vi "Arduino.vi"() -> ()   [LabVIEW 2015]
uses:
  <vilib>/MakerHub/LINX/Private/Type Defs/User Platform.ctl
  <vilib>/MakerHub/LINX/Private/Type Defs/Interface.ctl
  <vilib>/MakerHub/LINX/Public/Peripherals/PWM/Set Duty Cycle 1 Chan.vi
  <vilib>/MakerHub/LINX/LMH-LINX.lvlib
  <vilib>/MakerHub/LINX/Public/Peripherals/Digital/Digital Write 1 Chan.vi
  <vilib>/MakerHub/LINX/Public/Peripherals/Analog/Analog Read 1 Chan.vi
panel:
  in  "Duty Cycle (0-1)":dbl(knob) scale=0.0..0.2
  out "Loop Rate (Hz) 2":u32
  out "Loop Rate (Hz)":u32
  in  "Serial Port":refnum<visa-resource-name>="N/A"
  in  "Interface":T1
  in  "Platform":T2
  out "Waveform Chart":dbl(graph)
  in  "stop":bool
  in  "PWM Channel":u8
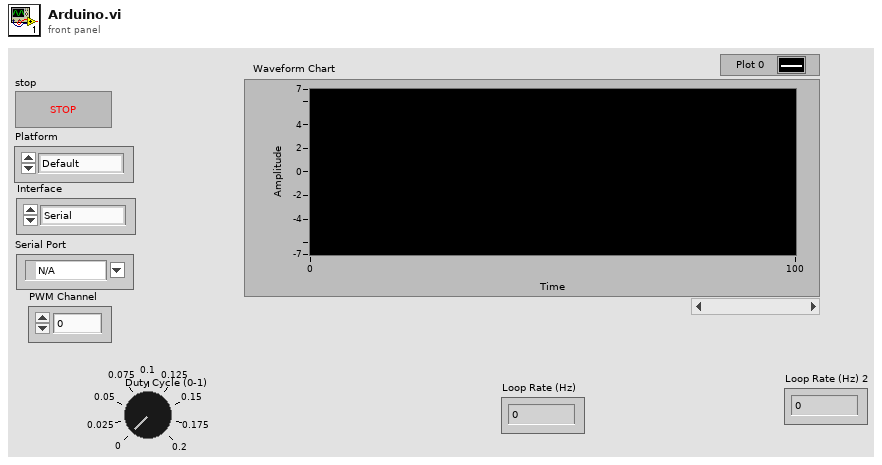
[diagram p1: front panel]
types:
  T1 = typedef "LMH-LINX.lvlib/Interface.ctl" = enum16{"Serial", "TCP"}
  T2 = typedef "LMH-LINX.lvlib/User Platform.ctl" = enum16{"Default", "LINX", "myRIO"}
  T3 = typedef "LMH-LINX.lvlib/LINX Ref.ctl" = cluster{"Platform":T4, "Interface":T1, "LINX Device Config":T5}
  T4 = typedef "LMH-LINX.lvlib/Platform.ctl" = enum16{"LINX", "myRIO"}
  T5 = typedef "LMH-LINX.lvlib/Device.lvlib/LINX Device Config.ctl" = cluster{"Interface":T1, "COM Port":refnum<visa-resource-name>, "TCP Configuration":T6, "Device Family":u8, "Device ID":u8, "Device Name":string, "TCP Ref":refnum<k5>, "Channels":T7}
  T6 = typedef "LMH-LINX.lvlib/Device.lvlib/TCP Config.ctl" = cluster{"IP Address":string, "Port":u16}
  T7 = typedef "LMH-LINX.lvlib/Channels.ctl" = cluster{"DI":u8[], "DO":u8[], "AI":u8[], "AO":u8[], "PWM":u8[], "QE":u8[], "UART":u8[], "I2C 2":u8[], "SPI":u8[], "CAN":u8[], "Servo":u8[], "AI Ref (V)":dbl, "AO Ref (V)":dbl, "AO Resolution (Bits)":u8}
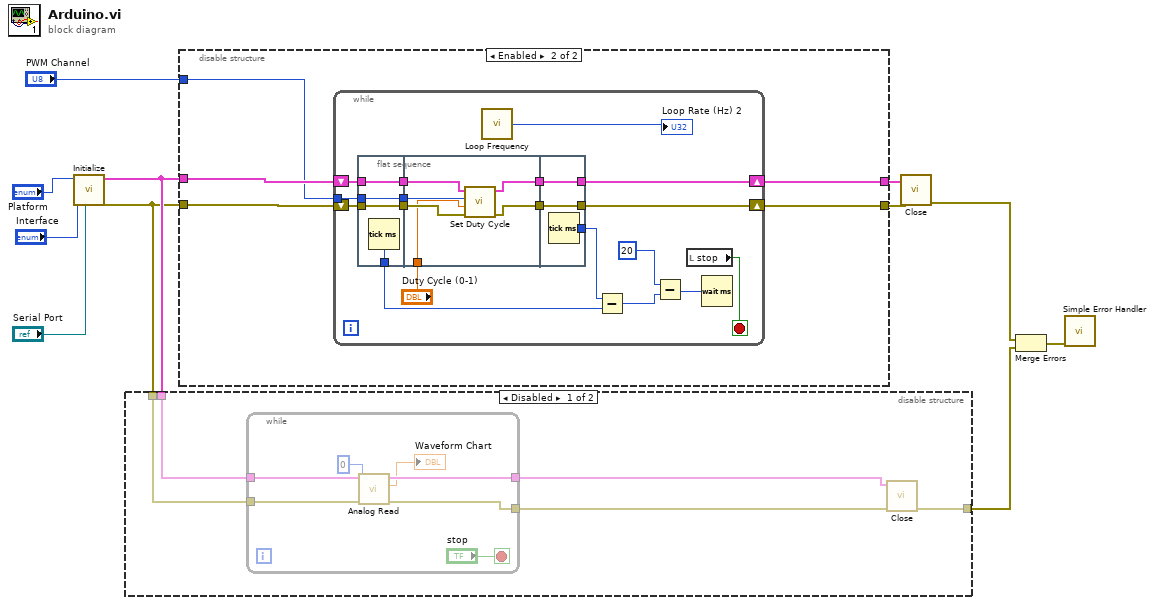
[diagram p0: block diagram]
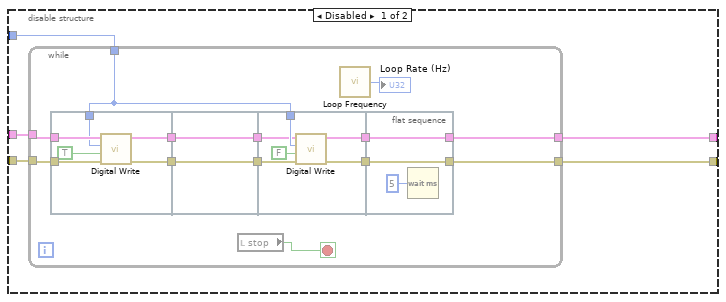
[diagram p3: hidden frame]
diagram:
  n1 = call <vilib>:"Initialize.vi"("Serial Port"="Serial Port", "Interface"="Interface", "Platform"="Platform") -> ("Error Out"=w5:errorcluster, "LINX Ref"=w8:T3)  [unwired: 6 in, 1 out]
  n2 = disable-structure shown="Disabled" {
    disable-tunnel: w8 -> [w15 _]
    disable-tunnel: [w14 _] -> w6
    disable-tunnel: w5 -> [w13 _]
    frame Disabled {
      n3 = while {
        tunnel: w15 -> [w23]
        tunnel: [w22] -> w16
        tunnel: w13 -> [w18]
        tunnel: [w17] -> w12
        stop <- "stop" stop-if-true
        n4 = call-poly <vilib>:"Analog Read.vi"("Error In"=w18, "Analog Channel"=u8 0, "LINX Resource"=w23) -> ("Error Out"=w17:errorcluster, "AI Value"=→"Waveform Chart":dbl, "LINX Resource"=w22:T3)  [unwired: 5 in, 1 out]
      }
      n5 = call <vilib>:"Close.vi"("Error In"=w12, "LINX Resource"=w16) -> ("Error Out"=w14:errorcluster)  [unwired: 8 in, 1 out]
    }
    frame Enabled {
    }
  }
  n6 = disable-structure shown="Enabled" {
    disable-tunnel: w8 -> [w28 w63]
    disable-tunnel: w5 -> [w27 w60]
    disable-tunnel: "PWM Channel" -> [w26 w61]
    disable-tunnel: [w24 w62] -> w3
    disable-tunnel: [w25 w59] -> w2
    frame Disabled {
      n7 = while {
        tunnel: w28 -> [w40]
        tunnel: w27 -> [w39]
        tunnel: w26 -> [w33]
        tunnel: [w32] -> w25
        tunnel: [w30] -> w24
        stop <- w41 stop-if-true
        n8 = flat-sequence {
          tunnel: w33 -> [w43]
          tunnel: [w46] -> w38
          tunnel: [w44] -> w37
          tunnel: w40 -> [w47]
          tunnel: w39 -> [w45]
          tunnel: w38 -> [w49]
          tunnel: w37 -> [w48]
          tunnel: [w49] -> w36
          tunnel: [w48] -> w35
          tunnel: w36 -> [w54]
          tunnel: w35 -> [w51]
          tunnel: w33 -> [w55]
          tunnel: [w52] -> w31
          tunnel: [w53] -> w29
          tunnel: [w58] -> w32
          tunnel: w31 -> [w58]
          tunnel: [w57] -> w30
          tunnel: w29 -> [w57]
          frame #0 {
            n9 = call-poly <vilib>:"Digital Write.vi"("Error In"=w45, "Output Value"=TRUE, "DO Channel"=w43, "LINX Resource"=w47) -> ("Error Out"=w44:errorcluster, "LINX Resource"=w46:T3)  [unwired: 6 in]
          }
          frame #1 {
          }
          frame #2 {
            n10 = call-poly <vilib>:"Digital Write.vi"("Error In"=w51, "Output Value"=FALSE, "DO Channel"=w55, "LINX Resource"=w54) -> ("Error Out"=w52:errorcluster, "LINX Resource"=w53:T3)  [unwired: 6 in]
          }
          frame #3 {
            n11 = Wait (ms)(milliseconds to wait=u32 5) -> ()  [unwired: 1 out]
          }
        }
        n12 = local read "stop"() -> (w41:bool)
        n13 = call <vilib>:"Loop Frequency.vi"() -> ("Loop Rate (Hz)"=→"Loop Rate (Hz)":u32)
      }
    }
    frame Enabled {
      n14 = while {
        tunnel: w61 -> [w79]
        shift-right: [w80] -> w62
        shift-left: w63 -> [w81]
        shift-right: [w77] -> w59
        shift-left: w60 -> [w78]
        stop <- w76 stop-if-true
        n15 = flat-sequence {
          tunnel: w78 -> [w83]
          tunnel: w79 -> [w84]
          tunnel: w81 -> [w85]
          tunnel: [w85] -> w74
          tunnel: [w84] -> w73
          tunnel: [w83] -> w72
          tunnel: [w82] -> w68
          tunnel: w74 -> [w91]
          tunnel: w73 -> [w89]
          tunnel: w72 -> [w88]
          tunnel: [w90] -> w71
          tunnel: [w87] -> w70
          tunnel: "Duty Cycle (0-1)" -> [w86]
          tunnel: [w93] -> w77
          tunnel: [w94] -> w80
          tunnel: w71 -> [w94]
          tunnel: w70 -> [w93]
          tunnel: [w92] -> w69
          frame #0 {
            n16 = Tick Count (ms)() -> (millisecond timer value=w82:u32)
          }
          frame #1 {
            n17 = call-poly <vilib>:"Set Duty Cycle.vi"("Error In"=w88, "Duty Cycle (0-1)"=w86, "PWM Channel"=w89, "LINX Resource"=w91) -> ("Error Out"=w87:errorcluster, "LINX Resource"=w90:T3)  [unwired: 6 in]
          }
          frame #2 {
            n18 = Tick Count (ms)() -> (millisecond timer value=w92:u32)
          }
        }
        n19 = call <vilib>:"Loop Frequency.vi"() -> ("Loop Rate (Hz)"=→"Loop Rate (Hz) 2":u32)
        n20 = Subtract(x=w69, y=w68) -> (x-y=w66:u32)
        n21 = Subtract(x=20, y=w66) -> (x-y=w65:u32)
        n22 = local read "stop"() -> (w76:bool)
        n23 = Wait (ms)(milliseconds to wait=w65) -> ()  [unwired: 1 out]
      }
    }
  }
  n24 = call <vilib>:"Close.vi"("Error In"=w2, "LINX Resource"=w3) -> ("Error Out"=w7:errorcluster)  [unwired: 8 in, 1 out]
  n25 = Merge Errors(w7, w6) -> (w1:errorcluster)
  n26 = call <vilib>:"Simple Error Handler.vi"("error in (no error)"=w1) -> ()  [unwired: 4 in, 5 out]
